vi "Process Global.vi"() -> ()   [LabVIEW 2019]
panel:
  out "Image 2":T1(plugin-control)
  out "Image":T1(plugin-control)
  out "AI結果":bool[](array[boolean])
  out "AlarmCycleNo_S11":i16
  out "AlarmCycleNo_S4":i16
  out "AlarmCycleNo_S3":i16
  out "AlarmCycleNo_S2":i16
  out "S4Tool Action":bool[](array[boolean])
  out "S3Tool Action":bool[](array[boolean])
  out "S2Tool Action":bool[](array[boolean])
  out "Tool Initial OK":bool
  out "process cluster before auto":cluster{string[], i32[]}
  in  "Step Content before auto":string[][](array[string])
  in  "S3 Tool String Display":string
  in  "機種廠商代號":string
  in  "硬體版本":string
  in  "S2 Tool String Display":string
  in  "S4 Tool String Display":string
  in  "T1 Current00":dbl
  out "S4 NG":bool
  out "S4 OK":bool
  out "S3 NG":bool
  out "S3 OK":bool
  out "S2 NG":bool
  out "S2 OK":bool
  out "T2 Voltage":string
  out "T2 μA":dbl format="%#_6f"
  in  "Laser Data":dbl
  out "process cluster S4":cluster{string[], i32[]}
  out "process cluster S3":cluster{string[], i32[]}
  in  "Step ContentS3":string[][](array[string])
  in  "Step ContentS4":string[][](array[string])
  out "EngMeasureTab":cluster{"Table Control":string[][]}[](array[cluster])
  out "process cluster":cluster{string[], i32[]}
  in  "Step Content":string[][](array[string])
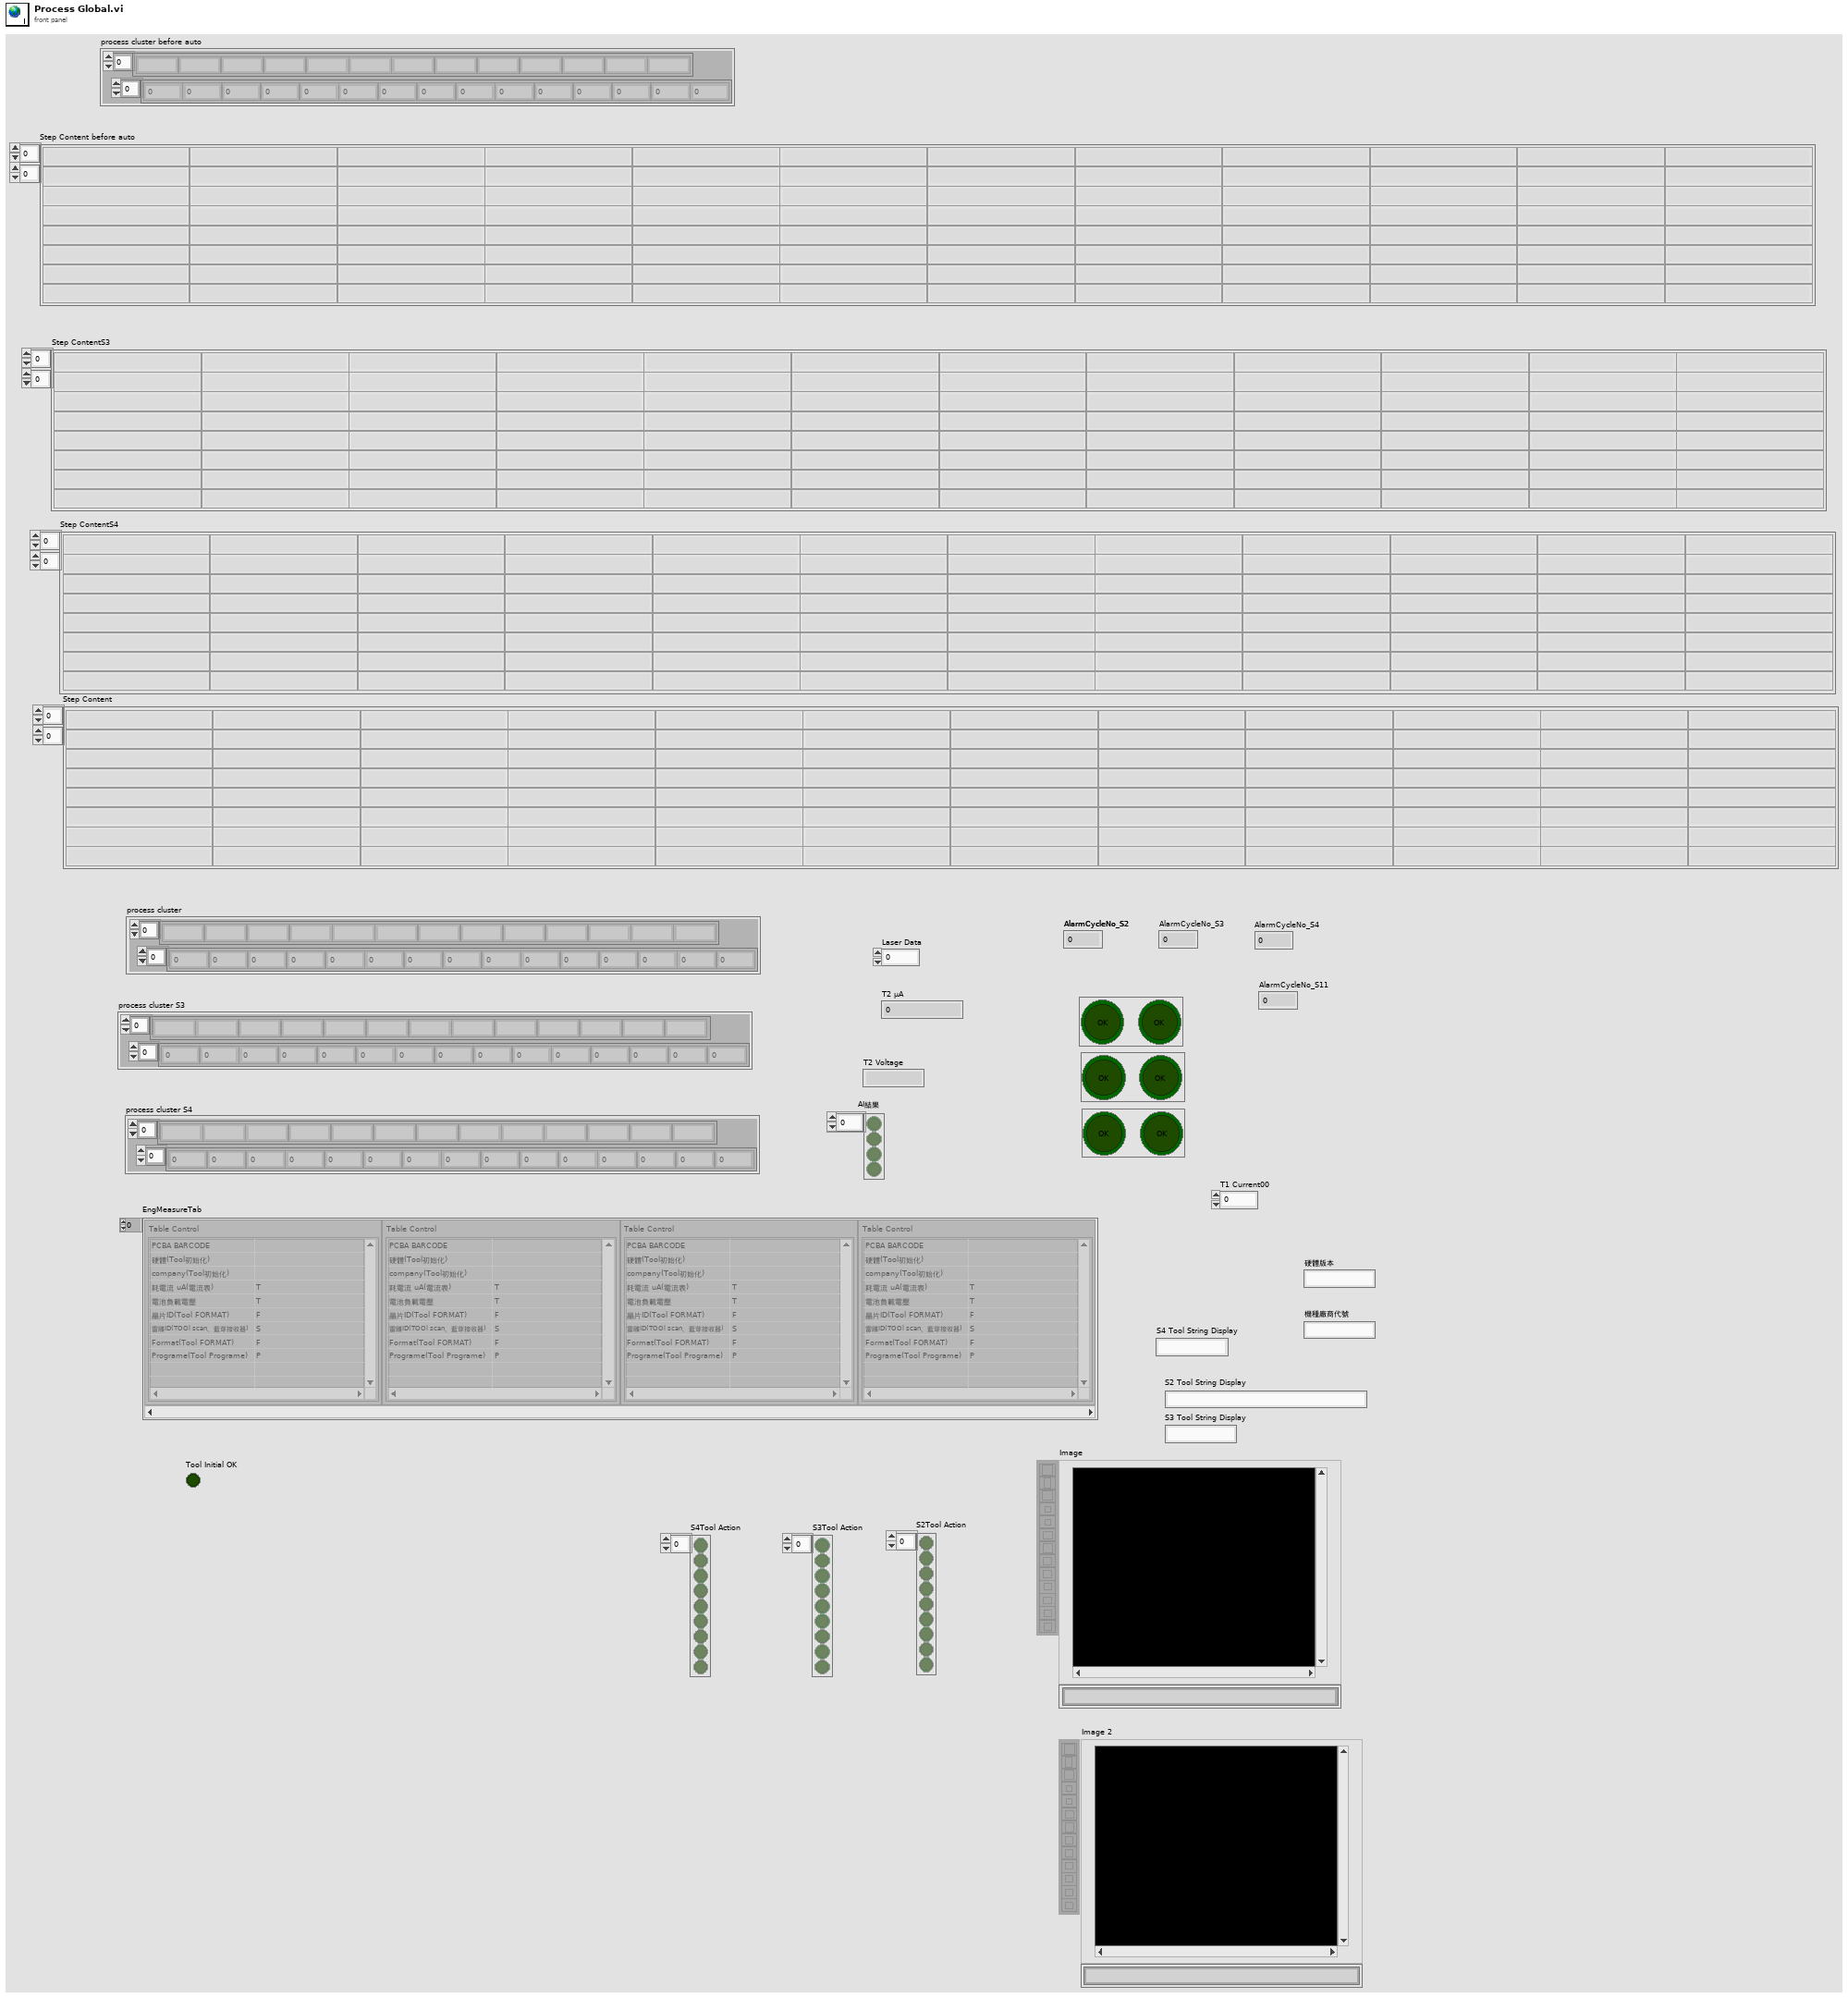
[diagram p1: front panel]
types:
  T1 = typedef "IMAQ Image.ctl" = refnum<image>
diagram:
